vi "New Parameter Message.vi"(8 "error in (no error)":errorcluster, 10 "New parameter":variant, 11 "Passive Hardware in":refnum<class "Passive Hardware.lvclass">) -> (0 "error out":errorcluster, 2 "New Parameter Message":T1, 3 "Passive Hardware out":refnum<class "Passive Hardware.lvclass">)   [LabVIEW 2020, in "RxnRover.lvlib" / "Passive Hardware.lvclass"]
doc: "Dynamic dispatch for each child controller type to provide it's proper message for setting a new parameter value (setpoint)."
uses:
  Passive Hardware.lvclass
  <userlib>/RxnRover/DynamicReentrant/src/Type Defs/Message.ctl
  Passive Hardware.lvclass/Passive Hardware.ctl
  <userlib>/RxnRover/DynamicReentrant/Dynamic Reentrant.lvlib
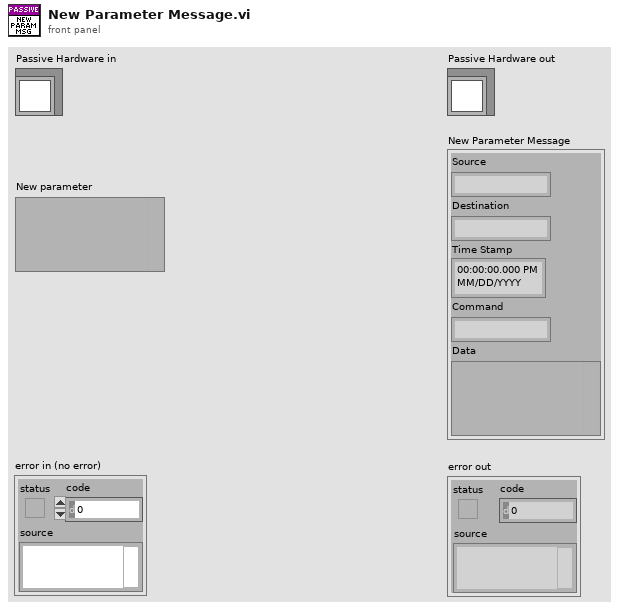
[diagram p1: front panel]
types:
  T1 = typedef "Dynamic Reentrant.lvlib/Message.ctl" = cluster{"Source":string, "Destination":string, "Time Stamp":timestamp, "Command":string, "Data":variant}
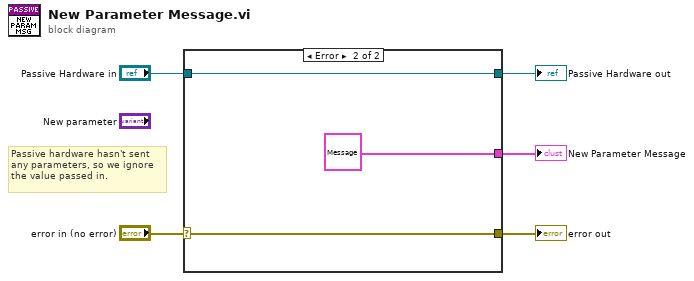
[diagram p0: block diagram]
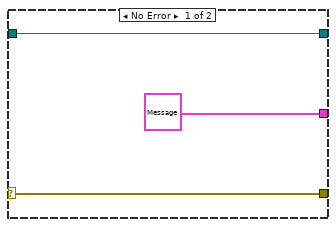
[diagram p2: hidden frame]
diagram:
  # "Passive hardware hasn't sent\nany parameters, so we ignore\nthe value passed in."
  n1 = case shown="Error" "error in (no error)" {
    selector: "error in (no error)" -> [w7 w11]
    tunnel: [w7 w11] -> w5
    tunnel: [w8 w10] -> w3
    tunnel: "Passive Hardware in" -> [w8 w10]
    tunnel: [T1 {"Source"="", "Destination"="", "Time Stamp"=timestamp(0 s since 1904-01-01), "Command"="New Parameter", "Data"=variant} ("Message") T1 {"Source"="", "Destination"="", "Time Stamp"=timestamp(0 s since 1904-01-01), "Command"="", "Data"=variant} ("Message")] -> w4
    frame No Error {
    }
    frame Error {
    }
  }
  "error out" <- w5
  "Passive Hardware out" <- w3
  "New Parameter Message" <- w4
